vi "OAT Convert Speed XY Graph to Waveform.vi"(0 "speed profile":T1 {"speed [RPM]" format="%.2f"; "time [s]" format="%.2f"}, 1 "reset? (F)":bool, 5 "analog tacho signal":waveform(dbl)={"t0"=timestamp(0 s since 1904-01-01), "dt"=0.0, "Y"=[]}, 7 "pulse/revolution (1)":i32, 9 "update rate (s)":dbl=0.01, 11 "error in (no error)":errorcluster, 12 "rotation direction":u16(ring) caption="rotation direction (CCW)" items=["CCW", "CW"]) -> (4 "waveform speed profile":waveform(dbl), 15 "error out":errorcluster)   [LabVIEW 2017, in "SoundVib_TachProcess.lvlib"]
doc: "Converts a speed profile XY graph to a waveform. This VI also attaches the information of the input speed profile XY graph and pulse-per-revolution to the output waveform."
uses:
  <vilib>/addons/Sound and Vibration/Order Analysis/Tach Process/SoundVib_TachProcess.lvlib
  <vilib>/addons/Sound and Vibration/Order Analysis/Tach Process/SubVIs/speed profile.ctl
  <vilib>/addons/_NISVFA/_Shared subVIs/Common/svc_Check for Waveform Parameter Continuity (no state).vi
  <vilib>/addons/_NISVFA/_Shared subVIs/Common/svc_Get SV Channel Info.vi
  <vilib>/addons/_NISVFA/_Shared subVIs/Common/svc_Engineering Units to Unit Label.vi
  <vilib>/addons/_NISVFA/_Shared subVIs/Common/svc_Unit Label to Engineering Units.vi
panel:
  in  "Waveform":waveform(dbl)={"t0"=timestamp(0 s since 1904-01-01), "dt"=0.0, "Y"=[]}
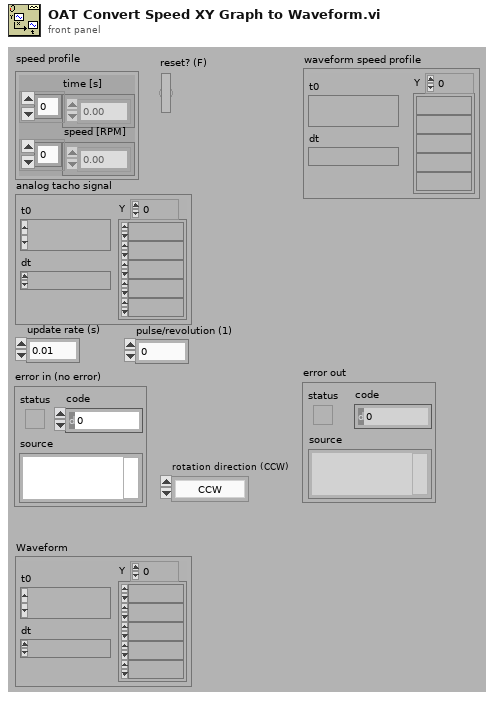
[diagram p1: front panel]
types:
  T1 = typedef "SoundVib_TachProcess.lvlib/speed profile.ctl" = cluster{"time [s]":dbl[], "speed [RPM]":dbl[]}
  T2 = cluster{"dt":bool, "t0 continuity":bool, "array length":bool, "channel info":bool, "name":bool}
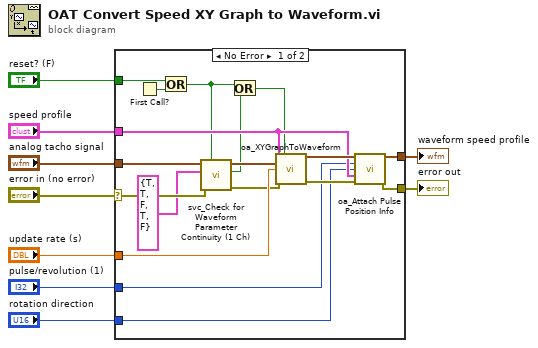
[diagram p0: block diagram]
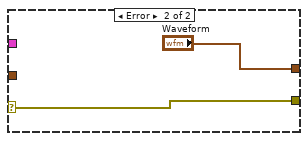
[diagram p2: hidden frame]
diagram:
  n1 = case shown="No Error" "error in (no error)" {
    selector: "error in (no error)" -> [w18 w28]
    tunnel: "analog tacho signal" -> [w20 _]
    tunnel: "update rate (s)" -> [w27 _]
    tunnel: "speed profile" -> [w24 _]
    tunnel: "pulse/revolution (1)" -> [w23 _]
    tunnel: "reset? (F)" -> [w15 _]
    tunnel: [w22 "Waveform"] -> w4
    tunnel: [w21 w28] -> w3
    tunnel: "rotation direction" -> [w10 _]
    frame No Error {
      n2 = First Call?() -> (First Call?: T/F=w14:bool)
      n3 = Or(x=w15, y=w14) -> (x .or. y?=w13:bool)
      n4 = call <vilib>:"svc_Check for Waveform Parameter Continuity (1 Ch).vi"("restart averaging (F)"=w13, "error in (no error)"=w18, "checks for channel parameter change"=T2 {"dt"=TRUE, "t0 continuity"=TRUE, "array length"=FALSE, "channel info"=TRUE, "name"=FALSE}, "scaled signal [EU]"=w20) -> ("error out"=w17:errorcluster, "waveform parameter changed"=w12:bool, "dup scaled signal [EU]"=w19:waveform(dbl))  [unwired: 2 in, 3 out]
      n5 = Or(x=w13, y=w12) -> (x .or. y?=w11:bool)
      n6 = call <vilib>:"oa_XYGraphToWaveform.vi"("input speed profile"=w24, "reset? (F)"=w11, "analog tacho signal"=w19, "update rate(s)"=w27, "error in (no error)"=w17) -> ("speed profile"=w26:waveform(dbl), "error out"=w25:errorcluster)  [unwired: 9 in]
      n7 = call <vilib>:"oa_Attach Pulse Position Info.vi"("speed profile signal input"=w26, "pulse/revolution (1)"=w23, "Rotation direction"=w10, "speed profile input"=w24, "error in (no error)"=w25) -> ("speed profile"=w22:waveform(dbl), "error out"=w21:errorcluster)  [unwired: 9 in]
    }
    frame Error {
    }
  }
  "error out" <- w3
  "waveform speed profile" <- w4
